vi "Update LCOS Image.vi"(0 "Images (Dest)":T1, 3 "error in":errorcluster) -> (6 "Images (Out)":T1, 9 "error out":errorcluster)   [LabVIEW 2011]
uses:
  LCOS Images.ctl
  <vilib>/vision/Image Controls.llb/IMAQ Image.ctl
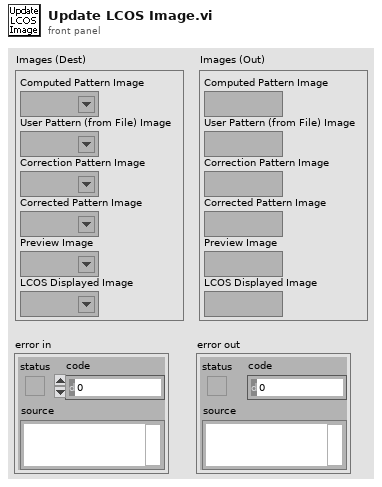
[diagram p1: front panel]
types:
  T1 = typedef "LCOS Images.ctl" = cluster{"Computed Pattern Image":T2, "User Pattern (from File) Image":T2, "Correction Pattern Image":T2, "Corrected Pattern Image":T2, "Preview Image":T2, "LCOS Displayed Image":T2}
  T2 = typedef "IMAQ Image.ctl" = refnum<image>
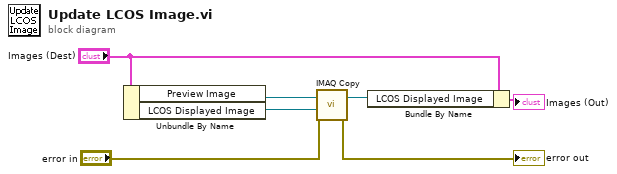
[diagram p0: block diagram]
diagram:
  n1 = Unbundle By Name("Images (Dest)") -> ("Preview Image"=w5:T2, "LCOS Displayed Image"=w3:T2)
  n2 = call "IMAQ Copy"("error in (no error)"="error in", "Image Dst"=w3, "Image Src"=w5) -> ("error out"=→"error out":errorcluster, "Image Dst Out"=w2:T2)  [unwired: 3 in]
  n3 = Bundle By Name(cluster="Images (Dest)", "LCOS Displayed Image"=w2) -> (→"Images (Out)":T1)
